vi "Acnet Past Value Reader.vi"(8 "error in (no error)":errorcluster, 10 "Time Stamp":timestamp, 11 "Device":string) -> (0 "error out":errorcluster, 3 "Reading":T1)   [LabVIEW 2013, in "Controls Log Monitor.lvlib"]
uses:
  MTA Shift Toolbox/Controls Log Monitor.lvlib
  <vilib>/httpClient/LabVIEWHTTPClient.lvlib
panel:
  out "headers":string
  out "body":string
  out "expanded url":string
  in  "url":string="http://www-ad.fnal.gov/cgi-bin/acl.pl?acl=read+${DEVICE}/src=dl:%22${TIME_STAMP}%22"
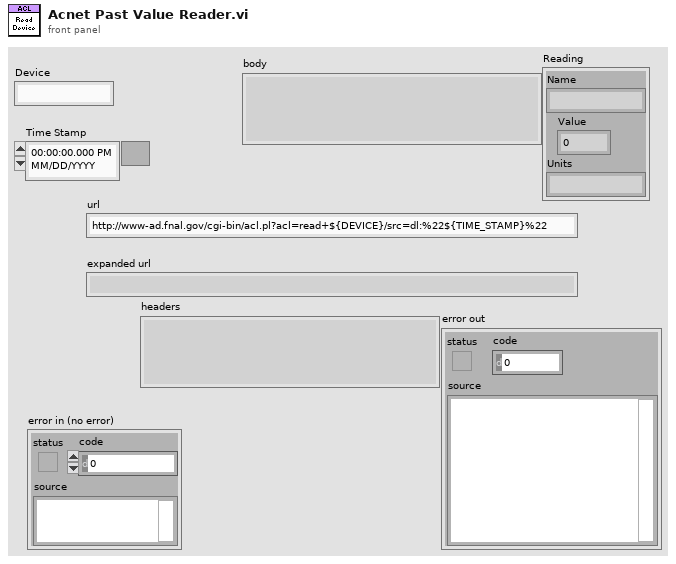
[diagram p1: front panel]
types:
  T1 = cluster{"Name":string, "Value":dbl, "Units":string}
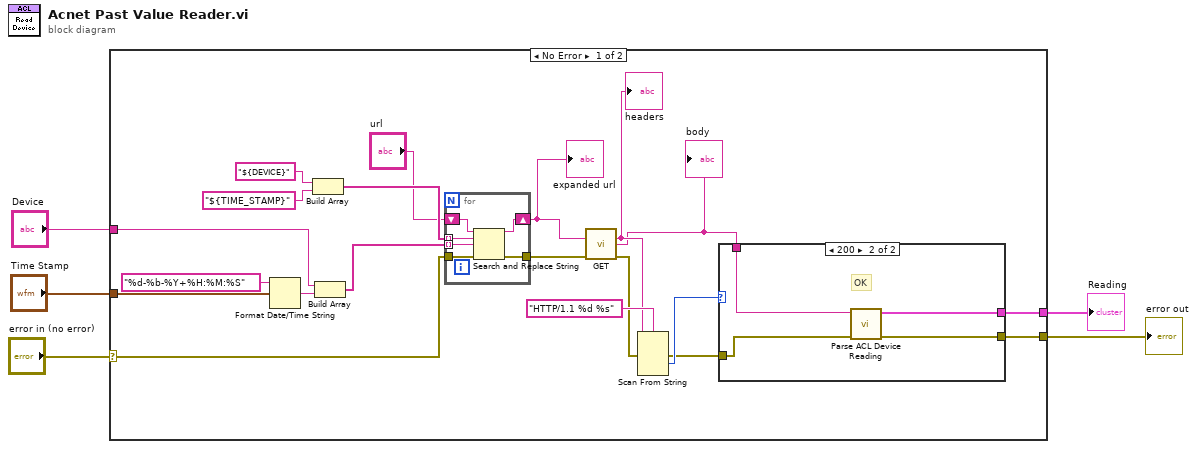
[diagram p0: block diagram]
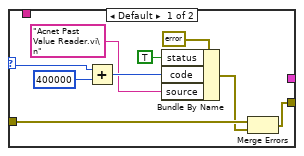
[diagram p2: hidden frame]
diagram:
  n1 = case shown="No Error" "error in (no error)" {
    selector: "error in (no error)" -> [w7 w45]
    tunnel: "Device" -> [w22 _]
    tunnel: "Time Stamp" -> [w21 _]
    tunnel: [w12 _] -> w3
    tunnel: [w11 w45] -> w2
    frame No Error {
      n2 = Format Date/Time String(time format string (%c)="%d-%b-%Y+%H:%M:%S", seconds (now)=w21) -> (date/time string=w18:string)  [unwired: 1 in]
      n3 = Build Array("${DEVICE}" ("search string"), "${TIME_STAMP}" ("element")) -> (w23:string[])
      n4 = Build Array(w22, w18) -> (w17:string[])
      n5 = for {
        tunnel: w23 -> [w44] mode=indexing
        tunnel: w17 -> [w43] mode=indexing
        tunnel: w7 -> [w42]
        tunnel: [w41] -> w10
        shift-right: [w40] -> w25
        shift-left: "url" -> [w39]
        n6 = Search and Replace String(input string=w39, search string=w44, replace string=w43, error in=w42) -> (result string=w40:string, error out=w41:errorcluster)  [unwired: 4 in, 2 out]
      }
      "expanded url" <- w25
      n7 = call <vilib>:"GET.vi"("url"=w25, "error in (no error)"=w10) -> ("headers"=w14:string, "body"=w6:string, "error out"=w9:errorcluster)  [unwired: 10 in, 1 out]
      "body" <- w6
      "headers" <- w14
      n8 = Scan From String(format string="HTTP/1.1 %d %s" ("headers"), input string=w14, error in=w9) -> (error out=w8:errorcluster, output 1=w13:i32)  [unwired: 4 in, 2 out]
      n9 = case shown="200" w13 {
        selector: w13 -> [w28 _]
        tunnel: w8 -> [w33 w36]
        tunnel: [w34 w35] -> w11
        tunnel: w6 -> [_ w38]
        tunnel: [_ w37] -> w12
        frame Default {
          n10 = Add(x=w28, y=400000 ("code")) -> (x+y=w27:i32)
          n11 = Bundle By Name(cluster=errorcluster {"status"=FALSE, "code"=0, "source"=""} ("error constant"), "status"=TRUE, "code"=w27, "source"="Acnet Past Value Reader.vi\n") -> (w30:errorcluster)
          n12 = Merge Errors(w33, w30) -> (w34:errorcluster)
        }
        frame 200 {
          # "OK"
          n13 = call "Parse ACL Device Reading.vi"("error in (no error)"=w36, "Reading String"=w38) -> ("error out"=w35:errorcluster, "Reading"=w37:T1)  [unwired: 8 in]
        }
      }
    }
    frame Error {
    }
  }
  "error out" <- w2
  "Reading" <- w3
